vi "get_top_level_VI_ref.vi"(8 "error in (no error)":errorcluster, 11 "GenericPlugin.lvclass in":refnum<class "GenericComponent.lvclass">) -> (0 "error out":errorcluster, 2 "top-level VI ref":refnum<vi>, 3 "GenericPlugin.lvclass out":refnum<class "GenericComponent.lvclass">)   [LabVIEW 2010, in "GenericComponent.lvclass"]
uses:
  GenericComponent.lvclass
  GenericComponent.lvclass/GenericComponent.ctl
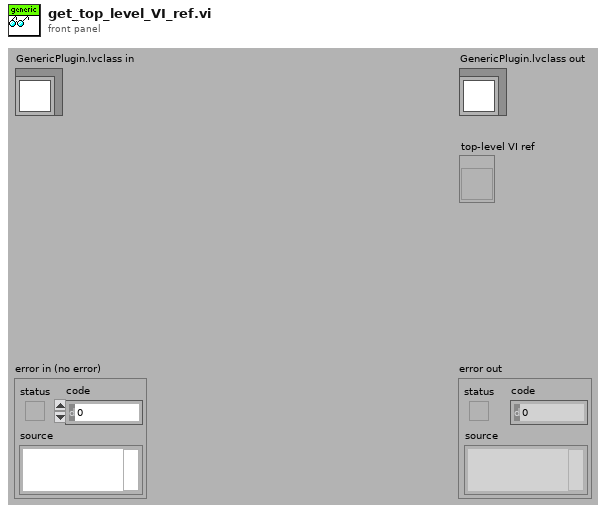
[diagram p1: front panel]
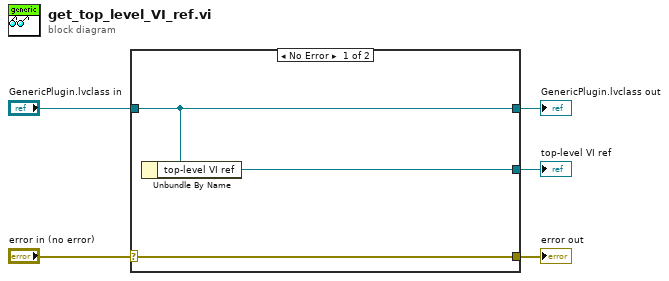
[diagram p0: block diagram]
diagram:
  n1 = case shown="No Error" "error in (no error)" {
    selector: "error in (no error)" -> [w8 w9]
    tunnel: [w8 w9] -> w4
    tunnel: [w7 w10] -> w2
    tunnel: "GenericPlugin.lvclass in" -> [w7 w10]
    tunnel: [w6 _] -> w1
    frame No Error {
      n2 = Unbundle By Name(w7) -> ("top-level VI ref"=w6:refnum<vi>)
    }
    frame Error {
    }
  }
  "error out" <- w4
  "GenericPlugin.lvclass out" <- w2
  "top-level VI ref" <- w1
